vi "Replace NaN by 0 (2D SGL).vi"(2 "Array in":sgl[][](array[numeric])) -> (7 "Array out":sgl[][](array[numeric]))   [LabVIEW 2021, in "Arrays.lvlib"]
uses:
  Arrays.lvlib
  df975b44-f6c5-4554-af30-980613d33749.vi
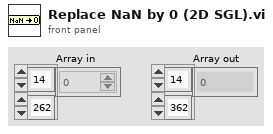
[diagram p1: front panel]
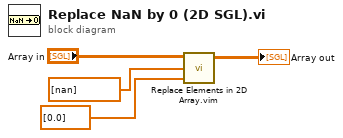
[diagram p0: block diagram]
diagram:
  n1 = call "Replace Elements in 2D Array.vim"("Array"="Array in", "Values to Replace"=sgl[] [nan], "Replacement Values"=sgl[] [0.0]) -> ("Modified Array"=→"Array out":sgl[][])  [unwired: 5 in, 1 out]
